vi "MGCC_FntStaMach_sitevisit_test.vi"() -> ()   [LabVIEW 2016]
panel:
  out "BusV_12":dbl
  out "BusV_10":dbl
  out "BusV_9":dbl
  out "BusV_8":dbl
  out "BusV_7":dbl
  out "BusV_6":dbl
  out "BusV_5":dbl
  out "BusV_4":dbl
  out "BusV_3":dbl
  out "BusV_2":dbl
  out "BusV_1":dbl
  out "MS_Binary_Status_OS2_8":bool
  out "MS_Binary_Status_OS2_7":bool
  out "MS_Binary_Status_OS2_6":bool
  out "MS_Binary_Status_OS2_5":bool
  out "MS_Binary_Status_OS2_4":bool
  out "MS_Binary_Status_OS2_3":bool
  out "MS_Binary_Status_OS2_2":bool
  out "MS_Binary_Status_OS2_1":bool
  in  "MS_Analog_Control_OS2_5":dbl
  in  "MS_Analog_Control_OS2_4":dbl
  in  "MS_Analog_Control_OS2_3":dbl
  in  "MS_Analog_Control_OS2_2":dbl
  in  "MS_Analog_Control_OS2_1":dbl
  out "MS_Analog_Status_OS2_19":dbl
  out "MS_Analog_Status_OS2_18":dbl
  out "MS_Analog_Status_OS2_17":dbl
  out "MS_Analog_Status_OS2_16":dbl
  out "MS_Analog_Status_OS2_15":dbl
  out "MS_Analog_Status_OS2_14":dbl
  out "MS_Analog_Status_OS2_13":dbl
  out "MS_Analog_Status_OS2_12":dbl
  out "MS_Analog_Status_OS2_11":dbl
  out "MS_Analog_Status_OS2_10":dbl
  out "MS_Analog_Status_OS2_9":dbl
  out "MS_Analog_Status_OS2_8":dbl
  out "MS_Analog_Status_OS2_7":dbl
  out "MS_Analog_Status_OS2_6":dbl
  out "MS_Analog_Status_OS2_5":dbl
  out "MS_Analog_Status_OS2_4":dbl
  out "MS_Analog_Status_OS2_3":dbl
  out "MS_Analog_Status_OS2_2":dbl
  out "MS_Analog_Status_OS2_1":dbl
  out "MS_Analog_Status_OS2_0":dbl
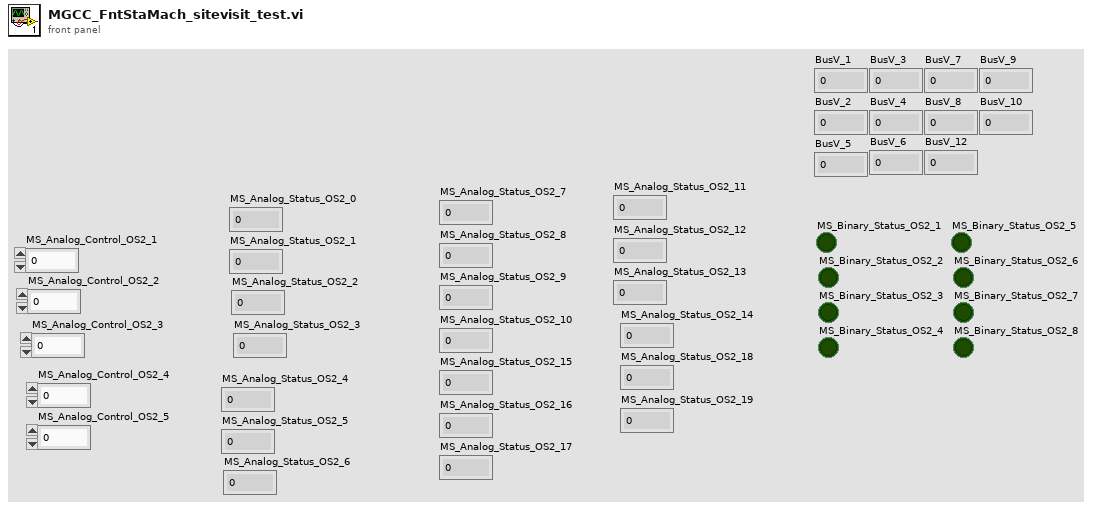
[diagram p1: front panel]
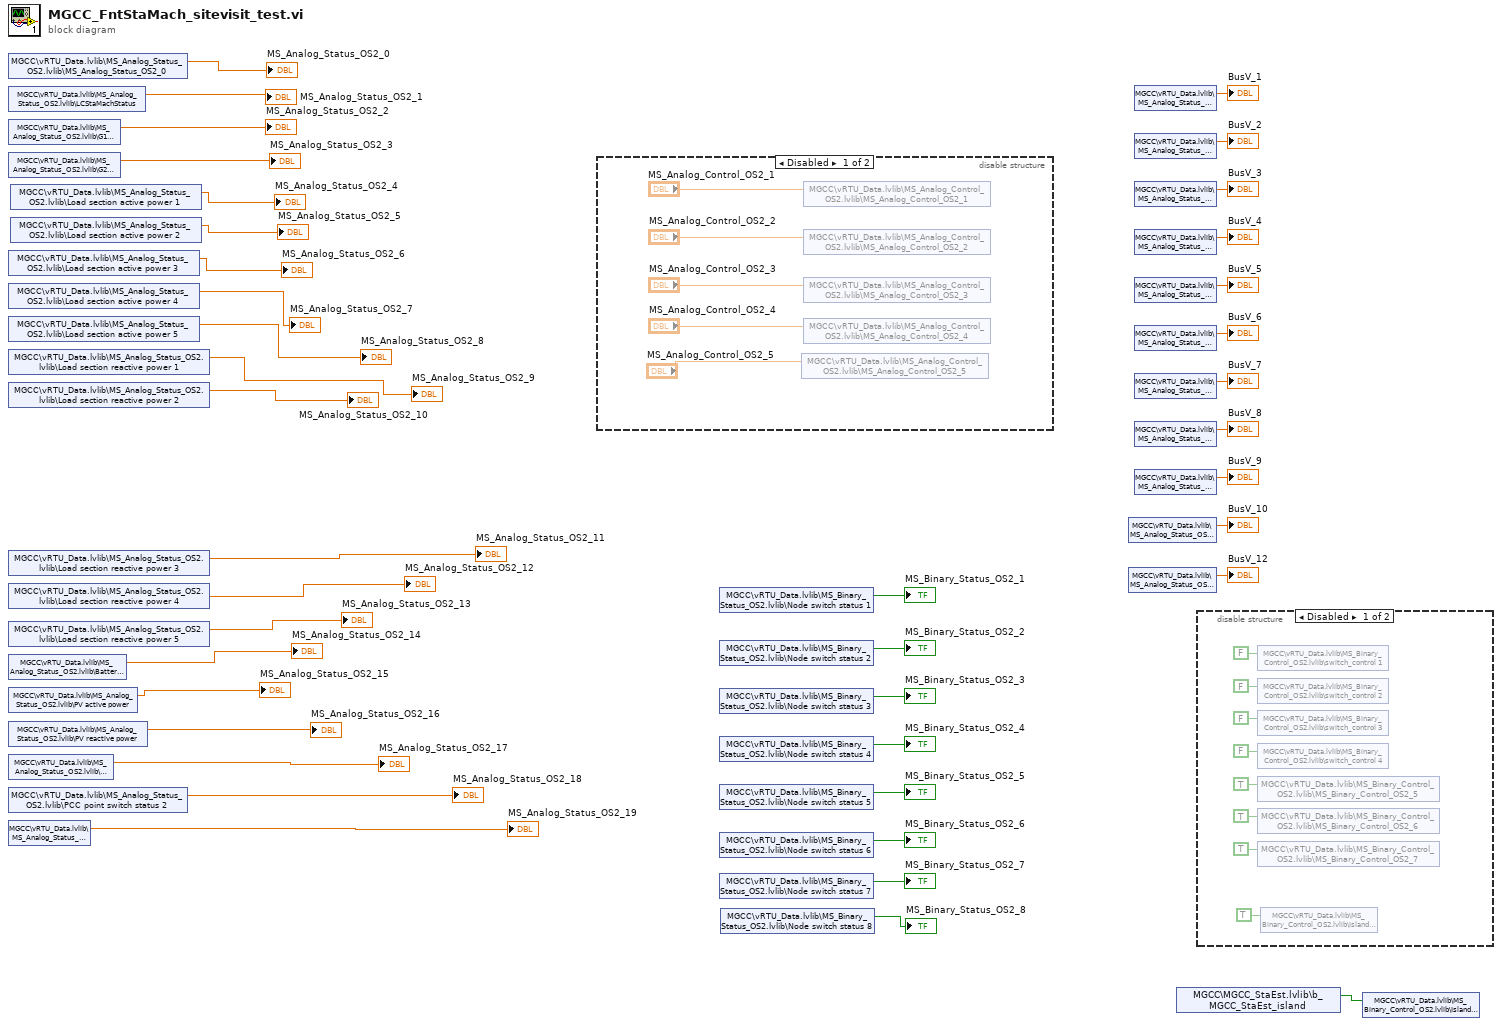
[diagram p0: block diagram]
diagram:
  n1 = shared-variable "MGCC\\vRTU_Data.lvlib\\MS_Analog_Status_OS2.lvlib\\MS_Analog_Status_OS2_0"() -> (→"MS_Analog_Status_OS2_0":dbl)  [unwired: 1 in, 1 out]
  n2 = shared-variable "MGCC\\vRTU_Data.lvlib\\MS_Analog_Status_OS2.lvlib\\LCStaMachStatus"() -> (→"MS_Analog_Status_OS2_1":dbl)  [unwired: 1 in, 1 out]
  n3 = shared-variable "MGCC\\vRTU_Data.lvlib\\MS_Analog_Status_OS2.lvlib\\G1 angle diff"() -> (→"MS_Analog_Status_OS2_2":dbl)  [unwired: 1 in, 1 out]
  n4 = shared-variable "MGCC\\vRTU_Data.lvlib\\MS_Analog_Status_OS2.lvlib\\G2 angle diff"() -> (→"MS_Analog_Status_OS2_3":dbl)  [unwired: 1 in, 1 out]
  n5 = shared-variable "MGCC\\vRTU_Data.lvlib\\MS_Analog_Status_OS2.lvlib\\Load section active power 3"() -> (→"MS_Analog_Status_OS2_6":dbl)  [unwired: 1 in, 1 out]
  n6 = shared-variable "MGCC\\vRTU_Data.lvlib\\MS_Analog_Status_OS2.lvlib\\Load section active power 4"() -> (→"MS_Analog_Status_OS2_7":dbl)  [unwired: 1 in, 1 out]
  n7 = shared-variable "MGCC\\vRTU_Data.lvlib\\MS_Analog_Status_OS2.lvlib\\Load section active power 5"() -> (→"MS_Analog_Status_OS2_8":dbl)  [unwired: 1 in, 1 out]
  n8 = shared-variable "MGCC\\vRTU_Data.lvlib\\MS_Analog_Status_OS2.lvlib\\Load section reactive power 1"() -> (→"MS_Analog_Status_OS2_9":dbl)  [unwired: 1 in, 1 out]
  n9 = shared-variable "MGCC\\vRTU_Data.lvlib\\MS_Analog_Status_OS2.lvlib\\Load section reactive power 2"() -> (→"MS_Analog_Status_OS2_10":dbl)  [unwired: 1 in, 1 out]
  n10 = shared-variable "MGCC\\vRTU_Data.lvlib\\MS_Analog_Status_OS2.lvlib\\Load section reactive power 3"() -> (→"MS_Analog_Status_OS2_11":dbl)  [unwired: 1 in, 1 out]
  n11 = shared-variable "MGCC\\vRTU_Data.lvlib\\MS_Analog_Status_OS2.lvlib\\Load section reactive power 4"() -> (→"MS_Analog_Status_OS2_12":dbl)  [unwired: 1 in, 1 out]
  n12 = shared-variable "MGCC\\vRTU_Data.lvlib\\MS_Analog_Status_OS2.lvlib\\Load section reactive power 5"() -> (→"MS_Analog_Status_OS2_13":dbl)  [unwired: 1 in, 1 out]
  n13 = shared-variable "MGCC\\vRTU_Data.lvlib\\MS_Analog_Status_OS2.lvlib\\Battery power"() -> (→"MS_Analog_Status_OS2_14":dbl)  [unwired: 1 in, 1 out]
  n14 = shared-variable "MGCC\\vRTU_Data.lvlib\\MS_Analog_Status_OS2.lvlib\\PV active power"() -> (→"MS_Analog_Status_OS2_15":dbl)  [unwired: 1 in, 1 out]
  n15 = shared-variable "MGCC\\vRTU_Data.lvlib\\MS_Analog_Status_OS2.lvlib\\PV reactive power"() -> (→"MS_Analog_Status_OS2_16":dbl)  [unwired: 1 in, 1 out]
  n16 = shared-variable "MGCC\\vRTU_Data.lvlib\\MS_Analog_Status_OS2.lvlib\\BatterySOC"() -> (→"MS_Analog_Status_OS2_17":dbl)  [unwired: 1 in, 1 out]
  n17 = shared-variable "MGCC\\vRTU_Data.lvlib\\MS_Analog_Status_OS2.lvlib\\PCC point switch status 2"() -> (→"MS_Analog_Status_OS2_18":dbl)  [unwired: 1 in, 1 out]
  n18 = shared-variable "MGCC\\vRTU_Data.lvlib\\MS_Analog_Status_OS2.lvlib\\BusV_1"() -> (→"MS_Analog_Status_OS2_19":dbl)  [unwired: 1 in, 1 out]
  n19 = shared-variable "MGCC\\vRTU_Data.lvlib\\MS_Analog_Status_OS2.lvlib\\Load section active power 1"() -> (→"MS_Analog_Status_OS2_4":dbl)  [unwired: 1 in, 1 out]
  n20 = shared-variable "MGCC\\vRTU_Data.lvlib\\MS_Analog_Status_OS2.lvlib\\Load section active power 2"() -> (→"MS_Analog_Status_OS2_5":dbl)  [unwired: 1 in, 1 out]
  n21 = disable-structure shown="Disabled" {
    frame Disabled {
      n22 = shared-variable "MGCC\\vRTU_Data.lvlib\\MS_Analog_Control_OS2.lvlib\\MS_Analog_Control_OS2_5"("MS_Analog_Control_OS2_5") -> ()  [unwired: 1 in, 1 out]
      n23 = shared-variable "MGCC\\vRTU_Data.lvlib\\MS_Analog_Control_OS2.lvlib\\MS_Analog_Control_OS2_1"("MS_Analog_Control_OS2_1") -> ()  [unwired: 1 in, 1 out]
      n24 = shared-variable "MGCC\\vRTU_Data.lvlib\\MS_Analog_Control_OS2.lvlib\\MS_Analog_Control_OS2_2"("MS_Analog_Control_OS2_2") -> ()  [unwired: 1 in, 1 out]
      n25 = shared-variable "MGCC\\vRTU_Data.lvlib\\MS_Analog_Control_OS2.lvlib\\MS_Analog_Control_OS2_3"("MS_Analog_Control_OS2_3") -> ()  [unwired: 1 in, 1 out]
      n26 = shared-variable "MGCC\\vRTU_Data.lvlib\\MS_Analog_Control_OS2.lvlib\\MS_Analog_Control_OS2_4"("MS_Analog_Control_OS2_4") -> ()  [unwired: 1 in, 1 out]
    }
    frame Enabled {
    }
  }
  n27 = shared-variable "MGCC\\vRTU_Data.lvlib\\MS_Binary_Status_OS2.lvlib\\Node switch status 1"() -> (→"MS_Binary_Status_OS2_1":bool)  [unwired: 1 in, 1 out]
  n28 = shared-variable "MGCC\\vRTU_Data.lvlib\\MS_Binary_Status_OS2.lvlib\\Node switch status 2"() -> (→"MS_Binary_Status_OS2_2":bool)  [unwired: 1 in, 1 out]
  n29 = shared-variable "MGCC\\vRTU_Data.lvlib\\MS_Binary_Status_OS2.lvlib\\Node switch status 3"() -> (→"MS_Binary_Status_OS2_3":bool)  [unwired: 1 in, 1 out]
  n30 = shared-variable "MGCC\\vRTU_Data.lvlib\\MS_Binary_Status_OS2.lvlib\\Node switch status 4"() -> (→"MS_Binary_Status_OS2_4":bool)  [unwired: 1 in, 1 out]
  n31 = shared-variable "MGCC\\vRTU_Data.lvlib\\MS_Binary_Status_OS2.lvlib\\Node switch status 5"() -> (→"MS_Binary_Status_OS2_5":bool)  [unwired: 1 in, 1 out]
  n32 = shared-variable "MGCC\\vRTU_Data.lvlib\\MS_Binary_Status_OS2.lvlib\\Node switch status 6"() -> (→"MS_Binary_Status_OS2_6":bool)  [unwired: 1 in, 1 out]
  n33 = shared-variable "MGCC\\vRTU_Data.lvlib\\MS_Binary_Status_OS2.lvlib\\Node switch status 7"() -> (→"MS_Binary_Status_OS2_7":bool)  [unwired: 1 in, 1 out]
  n34 = shared-variable "MGCC\\vRTU_Data.lvlib\\MS_Binary_Status_OS2.lvlib\\Node switch status 8"() -> (→"MS_Binary_Status_OS2_8":bool)  [unwired: 1 in, 1 out]
  n35 = shared-variable "MGCC\\vRTU_Data.lvlib\\MS_Analog_Status_OS2.lvlib\\BusV_10"() -> (→"BusV_10":dbl)  [unwired: 1 in, 1 out]
  n36 = shared-variable "MGCC\\vRTU_Data.lvlib\\MS_Analog_Status_OS2.lvlib\\BusV_11"() -> (→"BusV_12":dbl)  [unwired: 1 in, 1 out]
  n37 = shared-variable "MGCC\\vRTU_Data.lvlib\\MS_Analog_Status_OS2.lvlib\\BusV_1"() -> (→"BusV_1":dbl)  [unwired: 1 in, 1 out]
  n38 = shared-variable "MGCC\\vRTU_Data.lvlib\\MS_Analog_Status_OS2.lvlib\\BusV_2"() -> (→"BusV_2":dbl)  [unwired: 1 in, 1 out]
  n39 = shared-variable "MGCC\\vRTU_Data.lvlib\\MS_Analog_Status_OS2.lvlib\\BusV_3"() -> (→"BusV_3":dbl)  [unwired: 1 in, 1 out]
  n40 = shared-variable "MGCC\\vRTU_Data.lvlib\\MS_Analog_Status_OS2.lvlib\\BusV_4"() -> (→"BusV_4":dbl)  [unwired: 1 in, 1 out]
  n41 = shared-variable "MGCC\\vRTU_Data.lvlib\\MS_Analog_Status_OS2.lvlib\\BusV_5"() -> (→"BusV_5":dbl)  [unwired: 1 in, 1 out]
  n42 = shared-variable "MGCC\\vRTU_Data.lvlib\\MS_Analog_Status_OS2.lvlib\\BusV_6"() -> (→"BusV_6":dbl)  [unwired: 1 in, 1 out]
  n43 = shared-variable "MGCC\\vRTU_Data.lvlib\\MS_Analog_Status_OS2.lvlib\\BusV_7"() -> (→"BusV_7":dbl)  [unwired: 1 in, 1 out]
  n44 = shared-variable "MGCC\\vRTU_Data.lvlib\\MS_Analog_Status_OS2.lvlib\\BusV_8"() -> (→"BusV_8":dbl)  [unwired: 1 in, 1 out]
  n45 = shared-variable "MGCC\\vRTU_Data.lvlib\\MS_Analog_Status_OS2.lvlib\\BusV_9"() -> (→"BusV_9":dbl)  [unwired: 1 in, 1 out]
  n46 = shared-variable "MGCC\\MGCC_StaEst.lvlib\\b_MGCC_StaEst_island"() -> (w1:bool)  [unwired: 1 in, 1 out]
  n47 = disable-structure shown="Disabled" {
    frame Disabled {
      n48 = shared-variable "MGCC\\vRTU_Data.lvlib\\MS_Binary_Control_OS2.lvlib\\switch_control 1"(FALSE ("MS_Binary_Control_OS2_1")) -> ()  [unwired: 1 in, 1 out]
      n49 = shared-variable "MGCC\\vRTU_Data.lvlib\\MS_Binary_Control_OS2.lvlib\\switch_control 2"(FALSE ("MS_Binary_Control_OS2_2")) -> ()  [unwired: 1 in, 1 out]
      n50 = shared-variable "MGCC\\vRTU_Data.lvlib\\MS_Binary_Control_OS2.lvlib\\switch_control 3"(FALSE ("MS_Binary_Control_OS2_3")) -> ()  [unwired: 1 in, 1 out]
      n51 = shared-variable "MGCC\\vRTU_Data.lvlib\\MS_Binary_Control_OS2.lvlib\\switch_control 4"(FALSE ("MS_Binary_Control_OS2_4")) -> ()  [unwired: 1 in, 1 out]
      n52 = shared-variable "MGCC\\vRTU_Data.lvlib\\MS_Binary_Control_OS2.lvlib\\MS_Binary_Control_OS2_5"(TRUE ("MS_Binary_Control_OS2_5")) -> ()  [unwired: 1 in, 1 out]
      n53 = shared-variable "MGCC\\vRTU_Data.lvlib\\MS_Binary_Control_OS2.lvlib\\MS_Binary_Control_OS2_6"(TRUE ("MS_Binary_Control_OS2_6")) -> ()  [unwired: 1 in, 1 out]
      n54 = shared-variable "MGCC\\vRTU_Data.lvlib\\MS_Binary_Control_OS2.lvlib\\MS_Binary_Control_OS2_7"(TRUE ("MS_Binary_Control_OS2_7")) -> ()  [unwired: 1 in, 1 out]
      n55 = shared-variable "MGCC\\vRTU_Data.lvlib\\MS_Binary_Control_OS2.lvlib\\Island control"(TRUE ("MS_Binary_Control_OS2_8")) -> ()  [unwired: 1 in, 1 out]
    }
    frame Enabled {
    }
  }
  n56 = shared-variable "MGCC\\vRTU_Data.lvlib\\MS_Binary_Control_OS2.lvlib\\Island control"(w1) -> ()  [unwired: 1 in, 1 out]
